vi "HandleStateChange.vi"(8 "error in (no error)":errorcluster, 9 "UI State":T1=enum."Embedded", 10 "GUID":string, 11 "SMO.UI.MAUI in":refnum<class "SMO.UI.MAUI.lvclass">) -> (0 "error out":errorcluster, 3 "SMO.UI.MAUI out":refnum<class "SMO.UI.MAUI.lvclass">)   [LabVIEW 2019, in "SMO.UI.MAUI.lvclass"]
uses:
  SMO.UI.MAUI.lvclass
  <userlib>/LevyLab/Embedded UI/SMO.UI.Embedded/Typedefs/UI State.ctl
  SMO.UI.MAUI.lvclass/SMO.UI.MAUI.ctl
  <userlib>/LevyLab/Embedded UI/SMO.UI.Embedded/SMO.UI.Embedded.lvclass
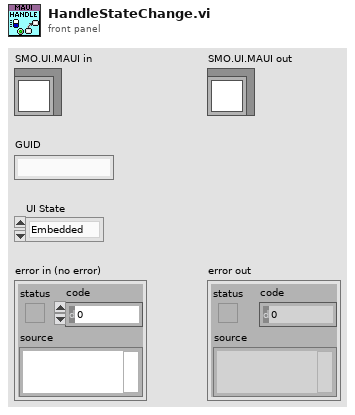
[diagram p1: front panel]
types:
  T1 = typedef "SMO.UI.Embedded.lvclass/UI State.ctl" = enum16{"unknown", "Opened", "Embedded", "Closed"}
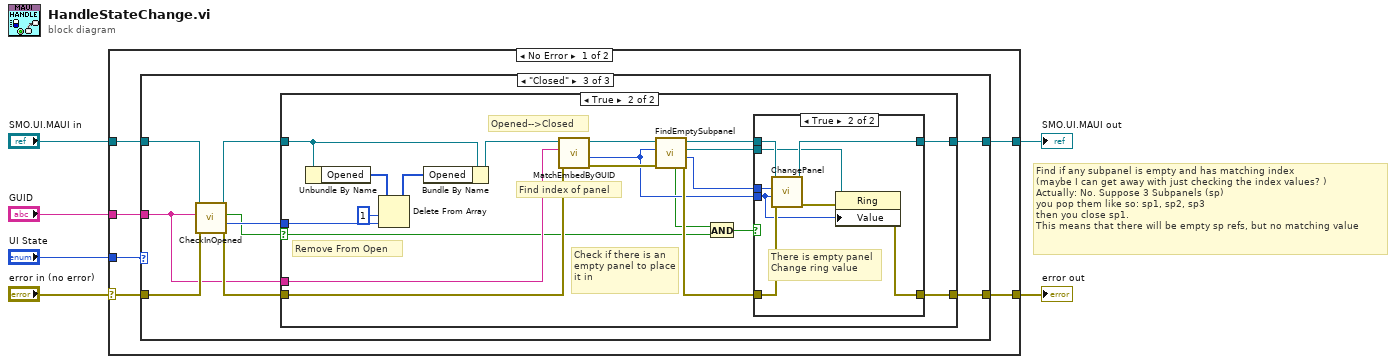
[diagram p0: block diagram]
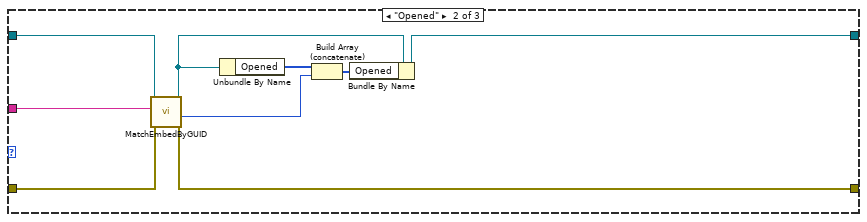
[diagram p3: hidden frame]
diagram:
  # "Find if any subpanel is empty and has matching index \n(maybe I can get away with just checking the index values? )\nActually: No. Suppose 3 Subpanels (sp)\nyou pop them like so: sp1, sp2, sp3\nthen you close sp1. \nThis means that there will be empty sp refs, but no matching value"
  n1 = case shown="No Error" "error in (no error)" {
    selector: "error in (no error)" -> [w11 w66]
    tunnel: [w12 w66] -> w5
    tunnel: [w10 w65] -> w3
    tunnel: "SMO.UI.MAUI in" -> [w9 w65]
    tunnel: "GUID" -> [w7 _]
    tunnel: "UI State" -> [w8 _]
    frame No Error {
      n2 = case shown="\"Closed\"" w8 {
        tunnel: [w13 w18 w28] -> w10
        tunnel: w9 -> [w13 w21 w29]
        tunnel: [w14 w23 w30] -> w12
        tunnel: w11 -> [w14 w22 w32]
        tunnel: w7 -> [_ w20 w27]
        frame Default {
        }
        frame "Opened" {
          n3 = call "MatchEmbedByGUID.vi"("error in (no error)"=w22, "GUID"=w20, "SMO.UI.MAUI in"=w21) -> ("error out"=w23:errorcluster, "Index"=w16:i32, "SMO.UI.MAUI out"=w15:refnum<class "SMO.UI.MAUI.lvclass">)  [unwired: 4 in, 2 out]
          n4 = Unbundle By Name(w15) -> ("Opened"=w19:i32[])
          n5 = Build Array (concatenate)(w19, w16) -> (w17:i32[])
          n6 = Bundle By Name(cluster=w15, "Opened"=w17) -> (w18:refnum<class "SMO.UI.MAUI.lvclass">)
        }
        frame "Closed" {
          n7 = call "CheckInOpened.vi"("error in (no error)"=w32, "GUID"=w27, "SMO.UI.MAUI in"=w29) -> ("error out"=w31:errorcluster, "Index"=w25:i32, "InOpened?"=w24:bool, "SMO.UI.MAUI out"=w26:refnum<class "SMO.UI.MAUI.lvclass">)  [unwired: 5 in]
          n8 = case shown="True" w24 {
            selector: w24 -> [_ w48]
            tunnel: w31 -> [w34 w54]
            tunnel: [w34 w51] -> w30
            tunnel: [w33 w46] -> w28
            tunnel: w26 -> [w33 w35]
            tunnel: w27 -> [_ w50]
            tunnel: w25 -> [_ w36]
            frame False {
              # "Embedded --> Closed\nDo nothing with Opened"
            }
            frame True {
              # "Check if there is an empty panel to place it in"
              # "Find index of panel"
              # "Remove From Open"
              # "Opened-->Closed"
              n9 = Unbundle By Name(w35) -> ("Opened"=w40:i32[])
              n10 = Delete From Array(array=w40, length=1, index=w36) -> (array with subset deleted=w38:i32[])  [unwired: 1 out]
              n11 = Bundle By Name(cluster=w35, "Opened"=w38) -> (w37:refnum<class "SMO.UI.MAUI.lvclass">)
              n12 = call "MatchEmbedByGUID.vi"("error in (no error)"=w54, "GUID"=w50, "SMO.UI.MAUI in"=w37) -> ("error out"=w53:errorcluster, "Index"=w45:i32, "SMO.UI.MAUI out"=w49:refnum<class "SMO.UI.MAUI.lvclass">)  [unwired: 4 in, 2 out]
              n13 = call "FindEmptySubpanel.vi"("error in (no error)"=w53, "Match Index"=w45, "SMO.UI.MAUI in"=w49) -> ("error out"=w52:errorcluster, "Subpanel Index"=w44:i32, "Ring Control"=w43:refnum<vi>, "SMO.UI.MAUI out"=w42:refnum<class "SMO.UI.MAUI.lvclass">, "Empty Subpanel Exists?"=w41:bool)  [unwired: 4 in]
              n14 = And(x=w41, y=w48) -> (x .and. y?=w47:bool)
              n15 = case shown="True" w47 {
                tunnel: w43 -> [_ w58]
                tunnel: w44 -> [_ w61]
                tunnel: w42 -> [w55 w59]
                tunnel: [w55 w60] -> w46
                tunnel: w45 -> [_ w57]
                tunnel: w52 -> [w56 w64]
                tunnel: [w56 w62] -> w51
                frame False {
                }
                frame True {
                  # "There is empty panel\nChange ring value"
                  n16 = call "ChangePanel.vi"("error in (no error)"=w64, "New Active Index"=w57, "Panel Index"=w61, "MAUI in"=w59) -> ("error out"=w63:errorcluster, "MAUI out"=w60:refnum<class "SMO.UI.MAUI.lvclass">)  [unwired: 6 in]
                  n17 = property class="Ring"(reference=w58, error in=w63, "Value"=w57) -> (error out=w62:errorcluster)  [unwired: 1 out]
                }
              }
            }
          }
        }
      }
    }
    frame Error {
    }
  }
  "error out" <- w5
  "SMO.UI.MAUI out" <- w3
